vi "di_continuous_lite.vi"() -> ()   [LabVIEW 2020]
uses:
  <vilib>/Waveform/DWDTOps.llb/DWDT Analog to Digital.vi
panel:
  out "DiFifoResidual":i32
  out "Rounds":i32
  in  "停止":bool
  out "error out":errorcluster caption="错误输出"
  out "数字波形图":digitalwaveform(graph)
  in  "SamplePeriod":u32=10000 caption="SamplePeriod (ns)"
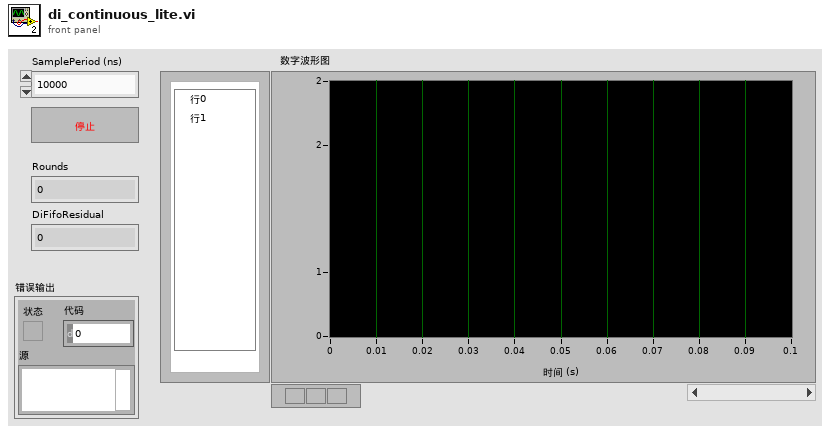
[diagram p1: front panel]
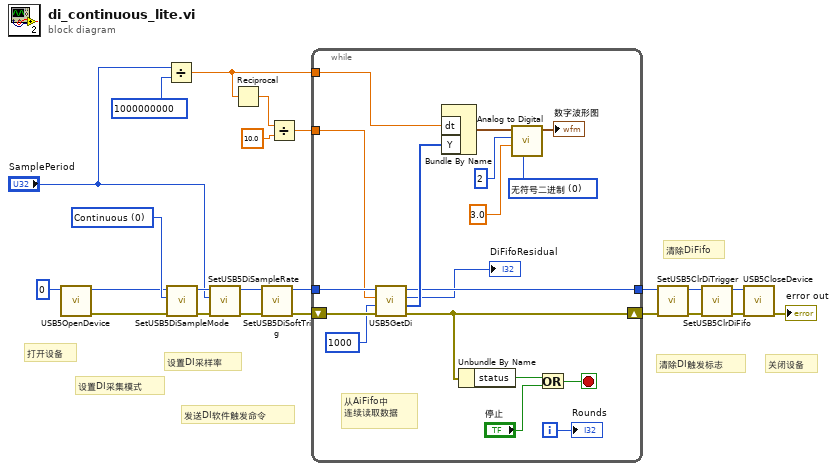
[diagram p0: block diagram]
diagram:
  w22 = u8 0 items=["Continuous", "OneShot"] ("DiSampleMode")
  # "关闭设备"
  # "清除DiFifo"
  # "清除DI触发标志"
  # "发送DI软件触发命令"
  # "设置DI采样率"
  # "设置DI采集模式"
  # "打开设备"
  n1 = call "USB5OpenDevice.vi"("DevIndex"=0) -> ("error out"=w2:errorcluster, "DevIndex Out"=w3:i32)  [unwired: 9 in]
  n2 = Divide(x="SamplePeriod", y=u32 1000000000) -> (x/y=w13:dbl)
  n3 = call "SetUSB5DiSampleMode.vi"("错误输入（无错误）"=w2, "DiSampleMode"=w22, "DevIndex"=w3) -> ("错误输出"=w21:errorcluster, "DevIndex Out"=w20:i32)  [unwired: 7 in]
  n4 = call "SetUSB5DiSampleRate.vi"("错误输入（无错误）"=w21, "SamplePeriod(ns)"="SamplePeriod", "DevIndex"=w20) -> ("错误输出"=w14:errorcluster, "DevIndex Out"=w15:i32)  [unwired: 7 in]
  n5 = Reciprocal(x=w13) -> (1/x=w12:dbl)
  n6 = call "SetUSB5DiSoftTrig.vi"("错误输入（无错误）"=w14, "DevIndex"=w15) -> ("错误输出"=w18:errorcluster, "DevIndex Out"=w19:i32)  [unwired: 8 in]
  n7 = Divide(x=w12, y=10.0) -> (x/y=w11:dbl)
  n8 = while {
    tunnel: w13 -> [w34]
    shift-right: [w27] -> w4
    shift-left: w18 -> [w40]
    tunnel: w11 -> [w29]
    tunnel: w19 -> [w41]
    tunnel: [w28] -> w5
    i -> [w26]
    stop <- w30 stop-if-true
    w36 = u16 0 items=["无符号二进制", "二进制偏移量", "二进制补码"] ("data format (offset binary)")
    # "从AiFifo中\n连续读取数据"
    n9 = call "USB5GetDi.vi"("错误输入（无错误）"=w40, "TimeOut"=1000, "Points"=w29, "DevIndex"=w41) -> ("错误输出"=w27:errorcluster, "Di"=w33:u8[], "DiFifoUsed"=→"DiFifoResidual":i32, "DevIndex Out"=w28:i32)  [unwired: 4 in]
    n10 = Bundle By Name("dt"=w34, "Y"=w33) -> (w35:waveform(u8))  [unwired: 1 in]
    n11 = Unbundle By Name(w27) -> ("status"=w32:bool)
    n12 = call-poly <vilib>:"Analog to Digital.vi"("data format (offset binary)"=w36, "full-scale range (pk-pk)"=3.0, "resolution (16 bit)"=2, "analog waveform"=w35) -> ("digital waveform"=→"数字波形图":digitalwaveform)  [unwired: 4 in, 3 out]
    n13 = Or(x=w32, y="停止") -> (x .or. y?=w30:bool)
    "Rounds" <- w26
  }
  n14 = call "SetUSB5ClrDiTrigger.vi"("错误输入（无错误）"=w4, "DevIndex"=w5) -> ("错误输出"=w7:errorcluster, "DevIndex Out"=w6:i32)  [unwired: 8 in]
  n15 = call "SetUSB5ClrDiFifo.vi"("错误输入（无错误）"=w7, "DevIndex"=w6) -> ("错误输出"=w8:errorcluster, "DevIndex Out"=w9:i32)  [unwired: 8 in]
  n16 = call "USB5CloseDevice.vi"("错误输入（无错误）"=w8, "DevIndex"=w9) -> ("error out"=→"error out":errorcluster)  [unwired: 8 in, 1 out]
